vi "Save Settings to XML.vi"(8 "error in (no error)":T5 caption="entrée d'erreur (pas d'erreur)", 11 "Paramètres":T1={"Configuration du matériel"={"Refnum de matériel <À remplacer>"="", "Type de signal <À remplacer>"=enum."Sine Wave"}, "Configuration de l'enregistrement"={"Chemin de base du fichier journal"=path "", "Référence de fichier TDMS"=refnum}, "Cluster test"={"Numérique"=15.0, "Numérique 2"=0.0}, "Mode de longueur d'onde"={"Choix du mode"=TRUE}}) -> (0 "error out":T5 caption="sortie d'erreur")   [LabVIEW 2018, in "Settings.lvlib"]
doc: "Enregistre les données de configuration \"Spécifiées par l'utilisateur\" dans un fichier XML. Il est utilisé pour retenir les paramètres utilisateur d'une exécution à l'autre."
uses:
  Settings.lvlib
  <vilib>/Utility/xml.llb/Write to XML File(string).vi
  Acquisition/Hardware Configuration.ctl
  Acquisition/Acquisition.lvlib
  Logging/Logging Configuration.ctl
  Logging/Logging.lvlib
  Settings.ctl
  Acquisition/Signal Type.ctl
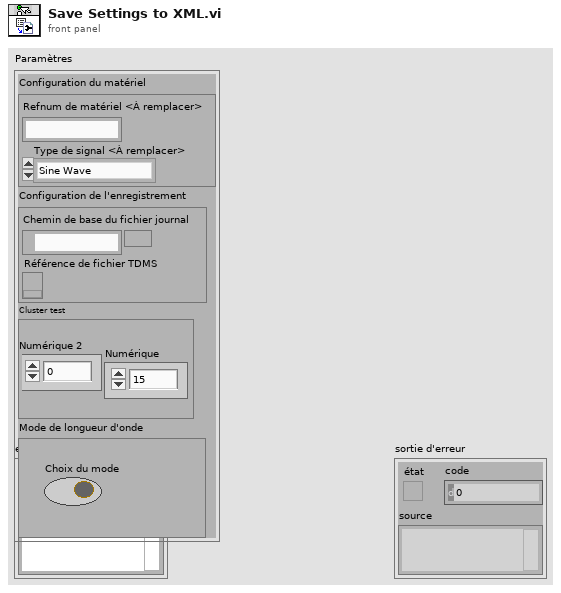
[diagram p1: front panel]
types:
  T1 = typedef "Settings.lvlib/Settings.ctl" = cluster{"Configuration du matériel":T2, "Configuration de l'enregistrement":T4, "Cluster test":cluster{"Numérique":dbl, "Numérique 2":dbl}, "Mode de longueur d'onde":cluster{"Choix du mode":bool}}
  T2 = typedef "Acquisition.lvlib/Hardware Configuration.ctl" = cluster{"Refnum de matériel <À remplacer>":string, "Type de signal <À remplacer>":T3}
  T3 = typedef "Acquisition.lvlib/Signal Type.ctl" = enum16{"Sine Wave", "Square with Noise", "Signal triangulaire", "Simulation DAQ"}
  T4 = typedef "Logging.lvlib/Logging Configuration.ctl" = cluster{"Chemin de base du fichier journal":path, "Référence de fichier TDMS":refnum<k34>}
  T5 = cluster{"état":bool, "code":i32, "source":string}
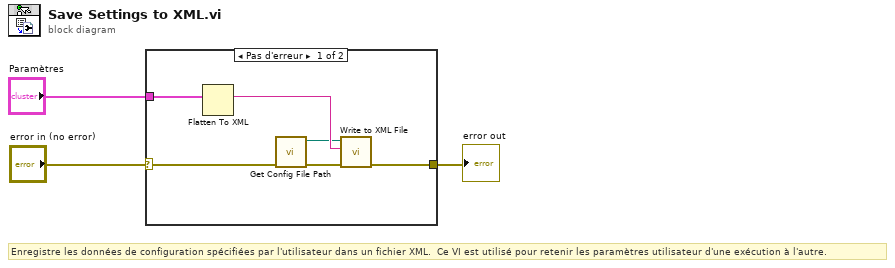
[diagram p0: block diagram]
diagram:
  # "Enregistre les données de configuration spécifiées par l'utilisateur dans un fichier XML.  Ce VI est utilisé pour retenir les paramètres utilisateur d'une exécution à l'autre."
  n1 = case shown="Pas d'erreur" "error in (no error)" {
    selector: "error in (no error)" -> [w5 w10]
    tunnel: [w7 w10] -> w2
    tunnel: "Paramètres" -> [w9 _]
    frame No Error {
      n2 = Flatten To XML(anything=w9) -> (xml string=w8:string)
      n3 = call "Get Config File Path.vi"("error in (no error)"=w5) -> ("error out"=w4:T5, "Chemin du fichier XML"=w6:path)  [unwired: 9 in]
      n4 = call-poly <vilib>:"Write to XML File.vi"("error in (no error)"=w4, "XML Input"=w8, "XML File Path"=w6) -> ("error out"=w7:errorcluster)  [unwired: 6 in, 2 out]
    }
    frame Error {
    }
  }
  "error out" <- w2
